vi "FileRichInfo2StringByTime.vi"(0 "file path (dialog if empty)":path caption="文件路径 （空时为对话框）", 1 "BeginTime":timestamp, 2 "EndTime":timestamp, 3 "总帧数":i32, 4 "文件类型":string="unknown", 5 "Language":u32) -> (8 "FileInfo":string)   [LabVIEW 2015]
panel:
  out "基时间秒 2":dbl format="%#.3f"
  out "基时间秒":dbl format="%#.3f"
  out "时间字符串 2":string
  out "时间字符串":string
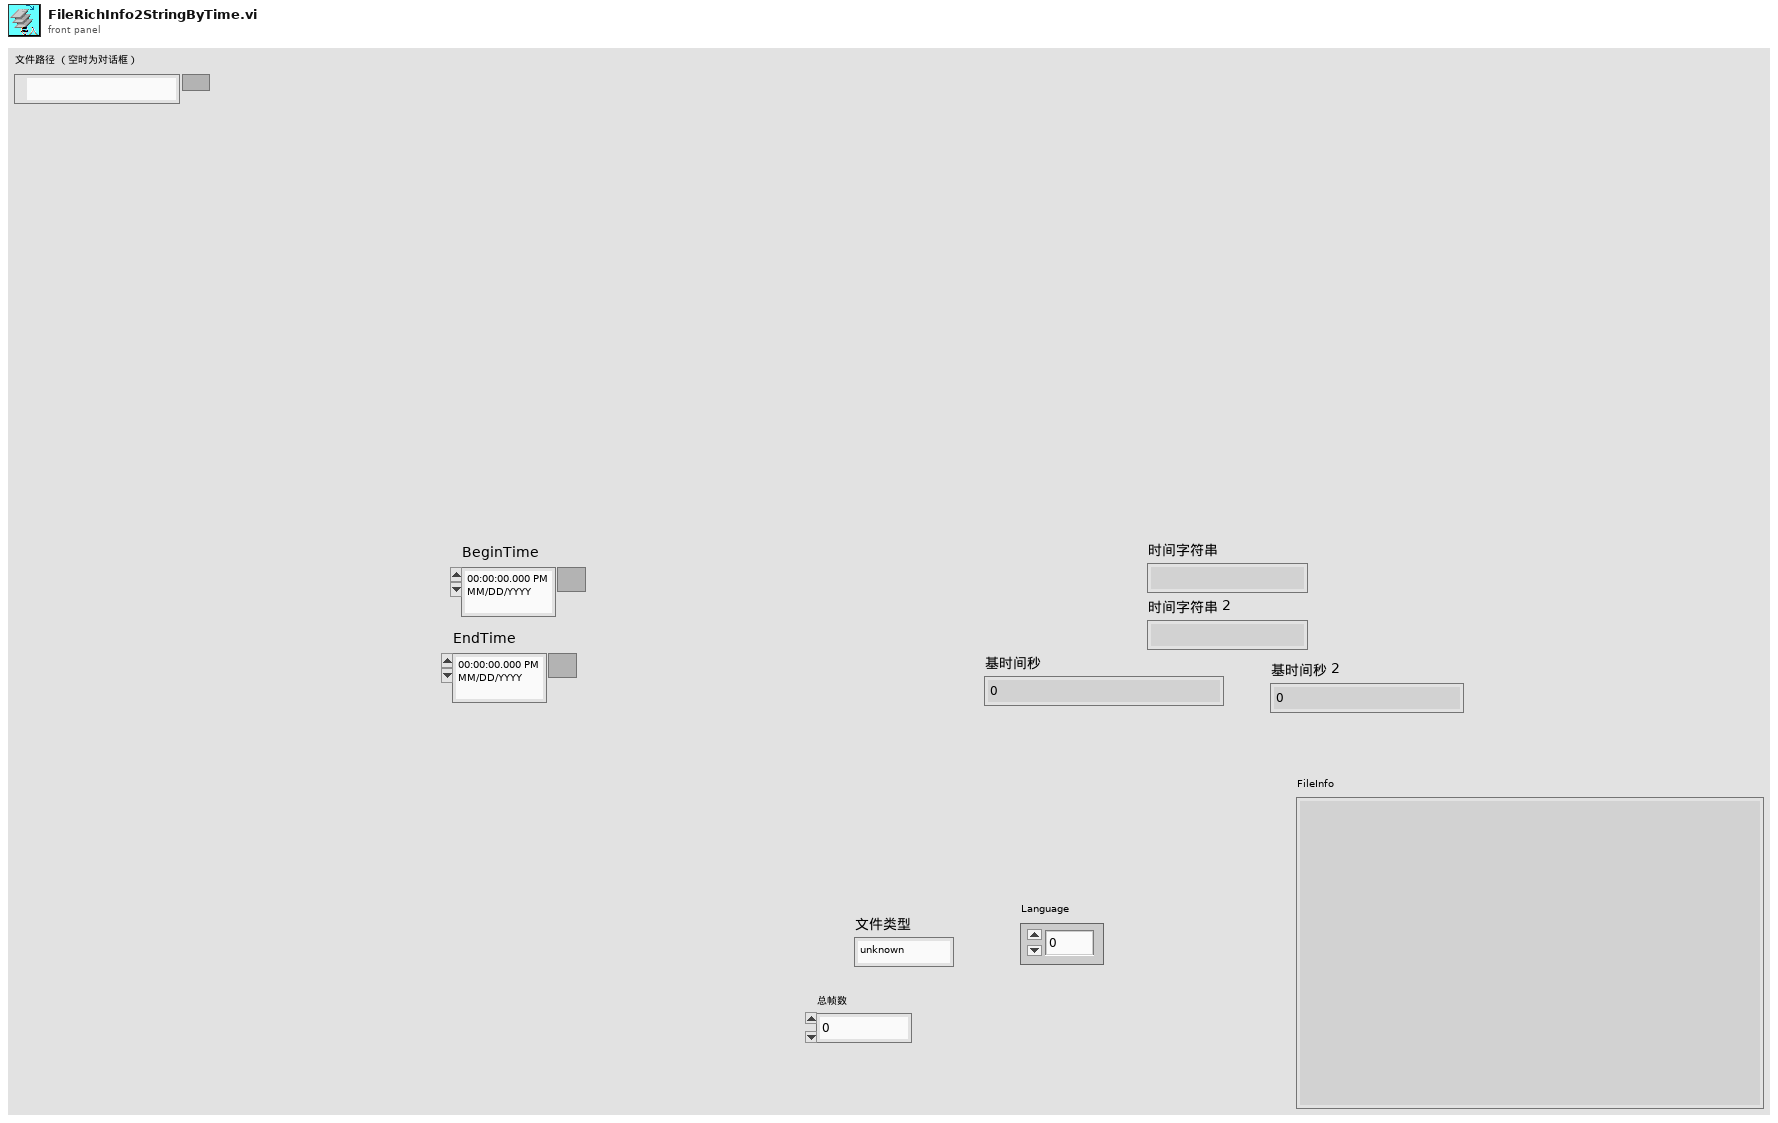
[diagram p1: front panel]
types:
  T1 = cluster{"基时间字符串":string, "基时间秒":dbl, "基时间标识":timestamp}
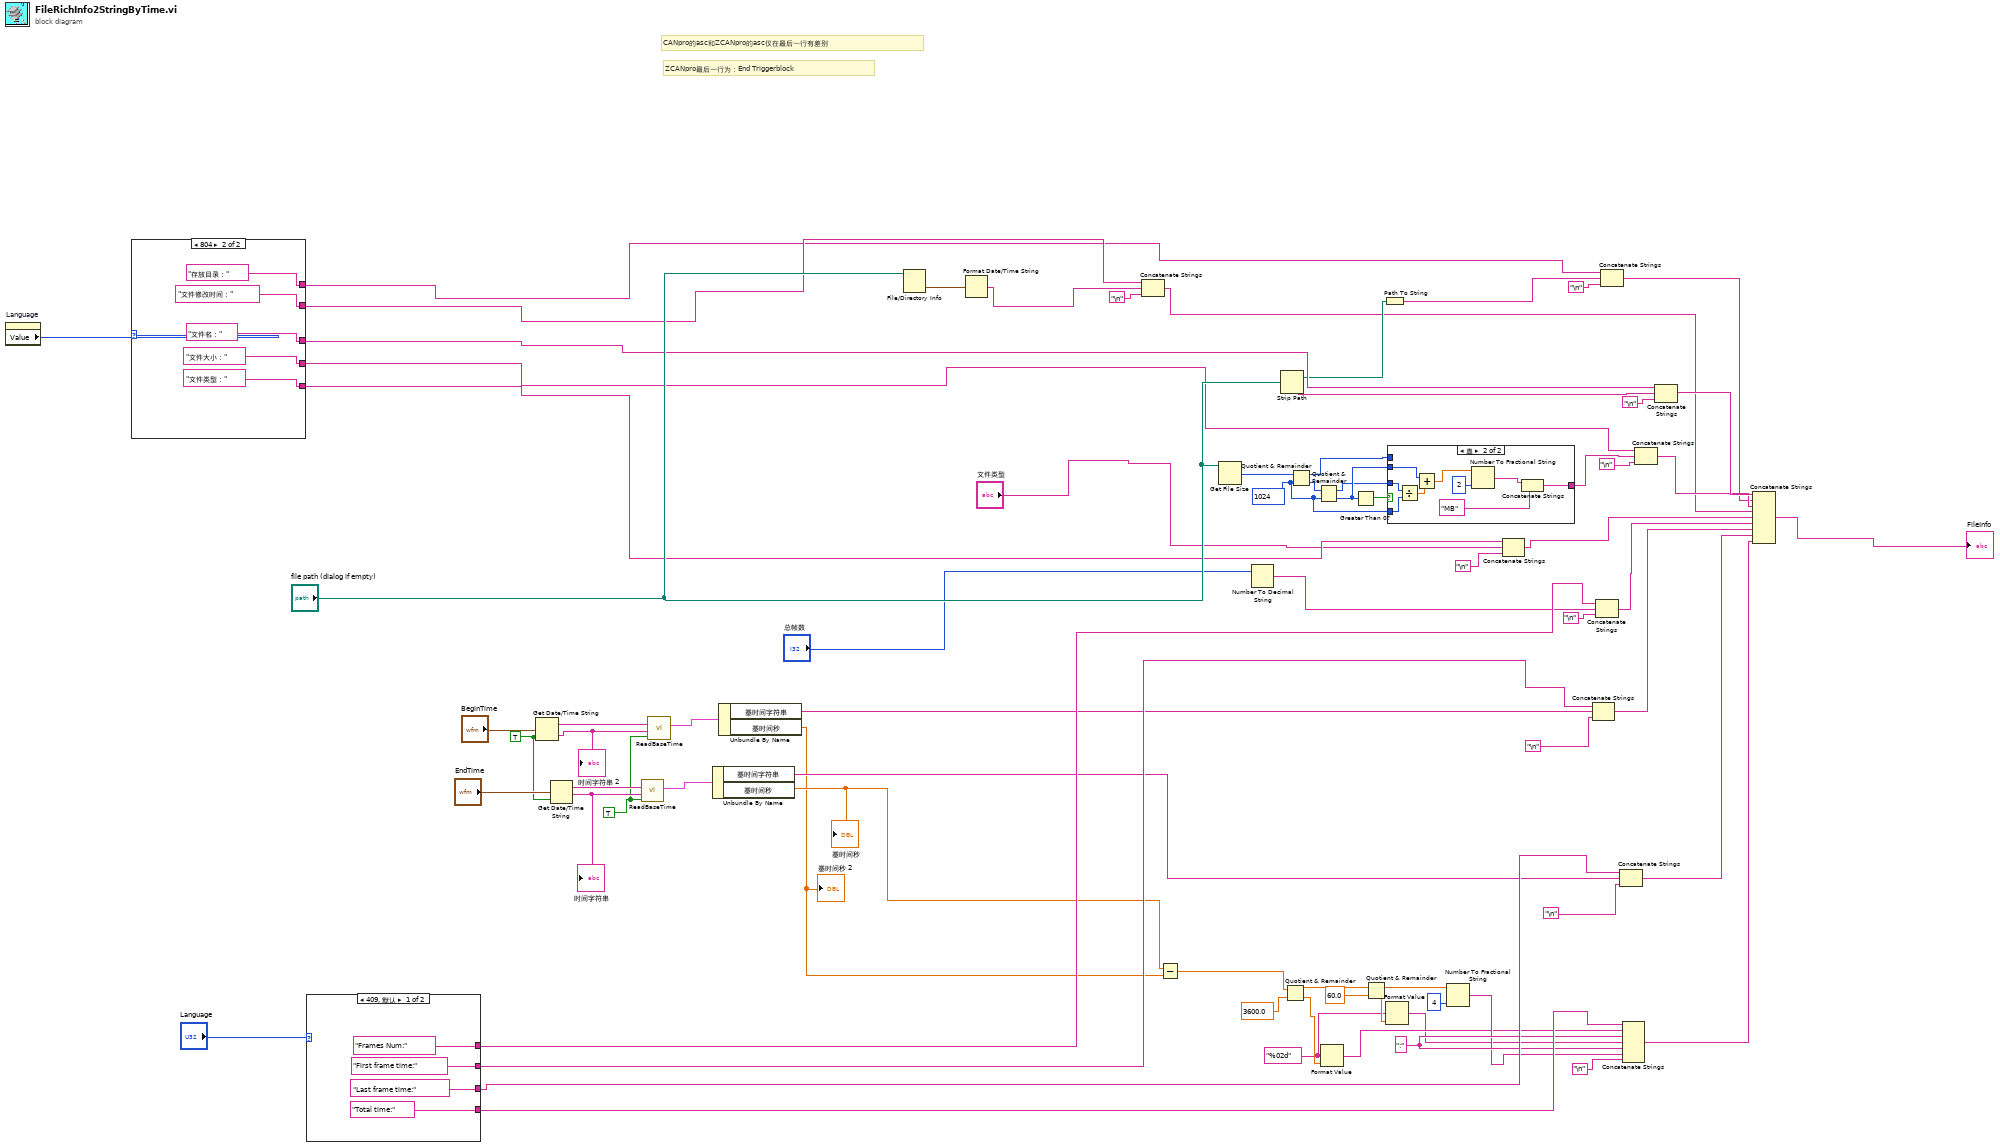
[diagram p0: block diagram]
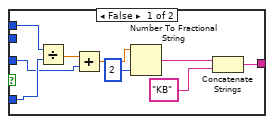
[diagram p2: hidden frame]
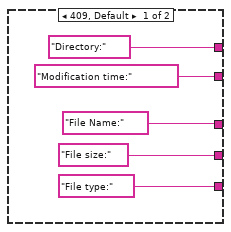
[diagram p3: hidden frame]
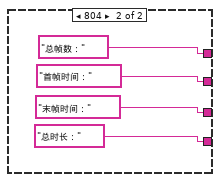
[diagram p4: hidden frame]
diagram:
  w1 = TRUE ("需要秒？(F)")
  w2 = TRUE ("文件时间？(F)")
  w31 = i64 1024 ("y")
  w48 = "%02d" ("格式字符串")
  w54 = ":"
  # "ZCANpro最后一行为：End Triggerblock"
  # "CANpro的asc和ZCANpro的asc仅在最后一行有差别"
  n1 = property on="Language" class="DigNum (严格)"() -> ("Value"=w71:u32)  [unwired: 2 in, 2 out]
  n2 = case shown="804" w71 {
    tunnel: ["Modification time:" "文件修改时间："] -> w70
    tunnel: ["Directory:" "存放目录："] -> w67
    tunnel: ["File Name:" "文件名："] -> w68
    tunnel: ["File size:" "文件大小："] -> w66
    tunnel: ["File type:" "文件类型："] -> w69
    frame 409, Default {
    }
    frame 804 {
    }
  }
  n3 = case shown="409, 默认" "Language" {
    tunnel: ["Total time:" "总时长："] -> w65
    tunnel: ["Last frame time:" "末帧时间："] -> w64
    tunnel: ["First frame time:" "首帧时间："] -> w63
    tunnel: ["Frames Num:" "总帧数："] -> w62
    frame 409, Default {
    }
    frame 804 {
    }
  }
  n4 = Get Date/Time String(seconds (now)="BeginTime", want seconds? (F)=w1) -> (date string=w6:string, time string=w7:string)  [unwired: 1 in]
  "时间字符串 2" <- w7
  n5 = Get Date/Time String(seconds (now)="EndTime", want seconds? (F)=w1) -> (date string=w14:string, time string=w13:string)  [unwired: 1 in]
  "时间字符串" <- w13
  n6 = call "ReadBaseTime.vi"("文件时间？(F)"=w2, "时间字符"=w13, "日期字符"=w14) -> ("基时间簇"=w16:T1)  [unwired: 6 in]
  n7 = call "ReadBaseTime.vi"("文件时间？(F)"=w2, "时间字符"=w7, "日期字符"=w6) -> ("基时间簇"=w5:T1)  [unwired: 6 in]
  n8 = Unbundle By Name(w16) -> ("基时间字符串"=w10:string, "基时间秒"=w15:dbl)
  "基时间秒" <- w15
  n9 = Unbundle By Name(w5) -> ("基时间字符串"=w4:string, "基时间秒"=w3:dbl)
  "基时间秒 2" <- w3
  n10 = File/Directory Info(path="file path (dialog if empty)") -> (last mod=w22:timestamp)  [unwired: 1 in, 6 out]
  n11 = Format Date/Time String(seconds (now)=w22) -> (date/time string=w20:string)  [unwired: 2 in]
  n12 = Concatenate Strings(w70, w20, "\n") -> (w19:string)
  n13 = Subtract(x=w15, y=w3) -> (x-y=w47:dbl)
  n14 = Get File Size(file="file path (dialog if empty)") -> (size (in bytes)=w34:i64)  [unwired: 1 in, 2 out]
  n15 = Number To Decimal String(number="总帧数") -> (decimal integer string=w37:string)  [unwired: 1 in]
  n16 = Strip Path(path="file path (dialog if empty)") -> (stripped path=w24:path, name=w44:string)
  n17 = Quotient & Remainder(x=w47, y=3600.0) -> (x-y*floor(x/y)=w58:dbl, floor(x/y)=w51:dbl)
  n18 = Quotient & Remainder(x=w34, y=w31) -> (x-y*floor(x/y)=w27:i64, floor(x/y)=w33:i64)
  n19 = Quotient & Remainder(x=w33, y=w31) -> (x-y*floor(x/y)=w29:i64, floor(x/y)=w30:i64)
  n20 = Format Value(format string=w48, value (0)=w51) -> (output string=w52:string)  [unwired: 1 in]
  n21 = Greater Than 0?(x=w30) -> (x > 0?=w32:bool)
  n22 = Quotient & Remainder(x=w58, y=60.0) -> (x-y*floor(x/y)=w56:dbl, floor(x/y)=w50:dbl)
  n23 = Path To String(path=w24) -> (string=w25:string)
  n24 = Format Value(format string=w48, value (0)=w50) -> (output string=w49:string)  [unwired: 1 in]
  n25 = case shown="真" w32 {
    tunnel: w31 -> [w98 w108]
    tunnel: w30 -> [_ w106]
    tunnel: w29 -> [w96 w109]
    tunnel: [w101 w104] -> w28
    tunnel: w27 -> [w99 _]
    frame False {
      n26 = Divide(x=w99, y=w98) -> (x/y=w97:dbl)
      n27 = Add(x=w97, y=w96) -> (x+y=w95:dbl)
      n28 = Number To Fractional String(number=w95, precision (6)=i16 2 ("精度(6)")) -> (F-format string=w93:string)  [unwired: 2 in]
      n29 = Concatenate Strings(w93, "KB" ("字符串")) -> (w101:string)
    }
    frame True {
      n30 = Divide(x=w109, y=w108) -> (x/y=w107:dbl)
      n31 = Add(x=w106, y=w107) -> (x+y=w105:dbl)
      n32 = Number To Fractional String(number=w105, precision (6)=i16 2 ("精度(6)")) -> (F-format string=w103:string)  [unwired: 2 in]
      n33 = Concatenate Strings(w103, "MB") -> (w104:string)
    }
  }
  n34 = Number To Fractional String(number=w56, precision (6)=i16 4 ("精度(6)")) -> (F-format string=w53:string)  [unwired: 2 in]
  n35 = Concatenate Strings(w69, "文件类型", "\n") -> (w41:string)
  n36 = Concatenate Strings(w63, w4, "\n") -> (w61:string)
  n37 = Concatenate Strings(w62, w37, "\n") -> (w38:string)
  n38 = Concatenate Strings(w67, w25, "\n") -> (w23:string)
  n39 = Concatenate Strings(w64, w10, "\n") -> (w60:string)
  n40 = Concatenate Strings(w65, w52, w54, w49, w54, w53, "\n") -> (w46:string)
  n41 = Concatenate Strings(w66, w28, "\n") -> (w35:string)
  n42 = Concatenate Strings(w68, w44, "\n") -> (w43:string)
  n43 = Concatenate Strings(w43, w23, w35, w19, w41, w38, w61, w60, w46) -> (→"FileInfo":string)
